vi "Translation stage.vi"() -> ()   [LabVIEW 2020]
panel:
  in  "Translation Stage Motor":refnum<k7>(container)
  in  "Number Of Translation Steps":i32=100
  out "Total Translation":sgl
  out "fAbsPosCh2":sgl
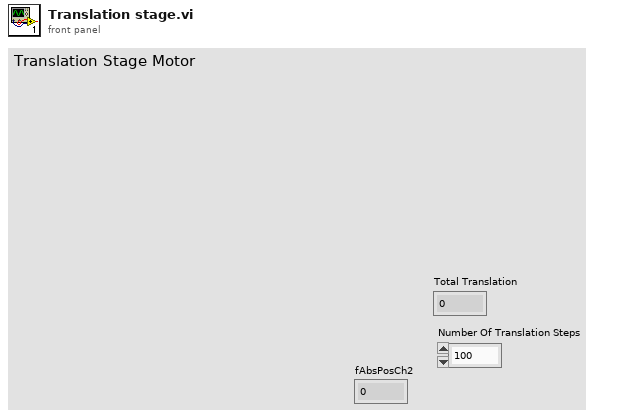
[diagram p1: front panel]
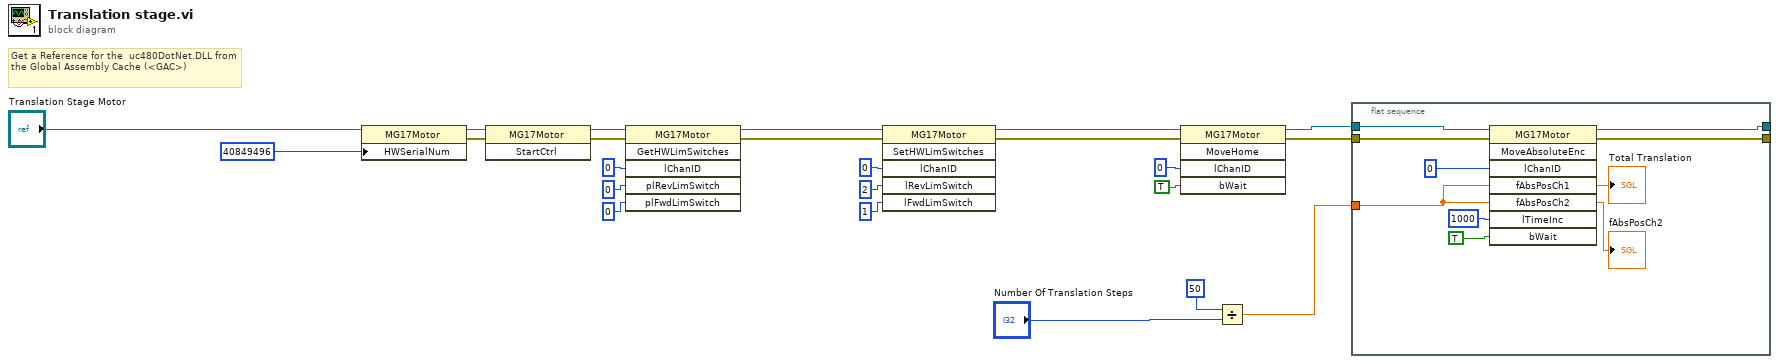
[diagram p0: block diagram]
diagram:
  # "Get a Reference for the  uc480DotNet.DLL from the Global Assembly Cache (<GAC>)"
  n1 = property class="MG17Motor"(reference="Translation Stage Motor", "HWSerialNum"=40849496) -> (reference out=w22:refnum<k7>, error out=w21:errorcluster)  [unwired: 1 in]
  n2 = invoke class="MG17Motor" method="StartCtrl"(reference=w22, error in=w21) -> (reference out=w20:refnum<k7>, error out=w19:errorcluster)  [unwired: 1 in, 1 out]
  n3 = invoke class="MG17Motor" method="GetHWLimSwitches"(reference=w20, error in=w19, "lChanID"=0, "plRevLimSwitch"=0, "plFwdLimSwitch"=0) -> (reference out=w8:refnum<k7>, error out=w9:errorcluster)  [unwired: 1 in, 4 out]
  n4 = invoke class="MG17Motor" method="SetHWLimSwitches"(reference=w8, error in=w9, "lChanID"=0, "lRevLimSwitch"=2 ("plRevLimSwitch"), "lFwdLimSwitch"=1 ("plFwdLimSwitch")) -> (reference out=w11:refnum<k7>, error out=w10:errorcluster)  [unwired: 1 in, 4 out]
  n5 = invoke class="MG17Motor" method="MoveHome"(reference=w11, error in=w10, "lChanID"=0, "bWait"=TRUE) -> (reference out=w4:refnum<k7>, error out=w3:errorcluster)  [unwired: 1 in, 3 out]
  n6 = Divide(x=50, y="Number Of Translation Steps") -> (x/y=w1:dbl)
  n7 = flat-sequence {
    tunnel: w4 -> [w32]
    tunnel: w3 -> [w31]
    tunnel: w1 -> [w24]
    tunnel: [w30] -> _
    tunnel: [w29] -> _
    frame #0 {
      n8 = invoke class="MG17Motor" method="MoveAbsoluteEnc"(reference=w32, error in=w31, "lChanID"=0, "fAbsPosCh1"=w24, "fAbsPosCh2"=w24, "lTimeInc"=1000, "bWait"=TRUE) -> (reference out=w30:refnum<k7>, error out=w29:errorcluster, "fAbsPosCh1"=→"Total Translation":sgl, "fAbsPosCh2"=→"fAbsPosCh2":sgl)  [unwired: 1 in, 4 out]
    }
  }
